vi "_Raise StatusBarTextChanged.vi"(4 "Display State In":T1, 5 "Event Data":cluster{"sender":refnum<k24>, "e":refnum<k24>}, 6 "Control Ref":refnum<k24>, 7 "Event Common Data":T2) -> ()   [LabVIEW 2020, in "WebView2 Control.xctl"]
uses:
  WebView2 Control.xctl
  E:/Labview/LV 2020/Libs/WebView2/LV-WebView2/Source/Libs/Microsoft.Web.WebView2.Core.dll
  Libs/Microsoft.Web.WebView2.Core.dll
  Events.ctl
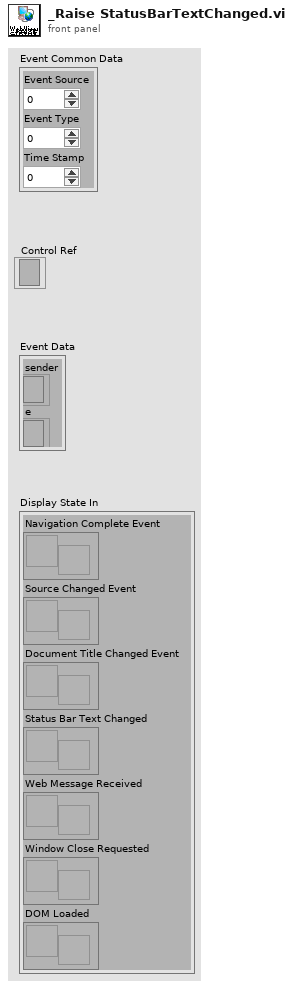
[diagram p1: front panel]
types:
  T1 = typedef "WebView2 Control.xctl/Events.ctl" = cluster{"Navigation Complete Event":refnum<user-event>, "Source Changed Event":refnum<user-event>, "Document Title Changed Event":refnum<user-event>, "Status Bar Text Changed":refnum<user-event>, "Web Message Received":refnum<user-event>, "Window Close Requested":refnum<user-event>, "DOM Loaded":refnum<user-event>}
  T2 = cluster{"Event Source":i32, "Event Type":u32, "Time Stamp":u32}
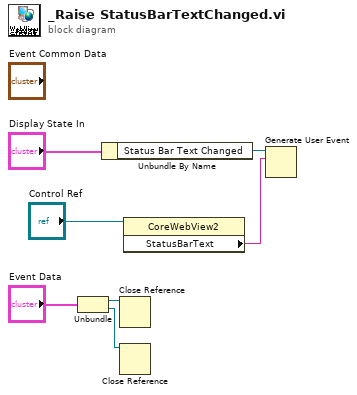
[diagram p0: block diagram]
diagram:
  n1 = Unbundle("Event Data") -> ("sender"=w2:refnum<k24>, "e"=w3:refnum<k24>)
  n2 = Unbundle By Name("Display State In") -> ("Status Bar Text Changed"=w5:refnum<user-event>)
  n3 = Close Reference(reference=w2) -> ()  [unwired: 1 in, 1 out]
  n4 = Close Reference(reference=w3) -> ()  [unwired: 1 in, 1 out]
  n5 = property class="CoreWebView2"(reference="Control Ref") -> ("StatusBarText"=w4:string)  [unwired: 1 in, 2 out]
  n6 = Generate User Event(user event=w5, event data cluster=w4) -> ()  [unwired: 2 in, 2 out]
